vi "Door Closed Interlock Value Change.vi"(8 "error in (no error)":errorcluster, 10 "Door Closed Interlock":bool, 11 "Doors Open in":refnum<class "Doors Open.lvclass">) -> (0 "error out":errorcluster, 3 "Doors Open out":refnum<class "Doors Open.lvclass">)   [LabVIEW 2020, in "Door Controller.lvlib" / "Doors Open.lvclass"]
uses:
  Doors Open.lvclass
  C:/Users/Thomas.McQuillan/Desktop/Elevator Door Control/Door Controller/Door Controller/Door Controller.lvclass
  Application/Application/Interlock Names.ctl
  Door Controller/Door Controller.lvclass
  Application/Application.lvlib
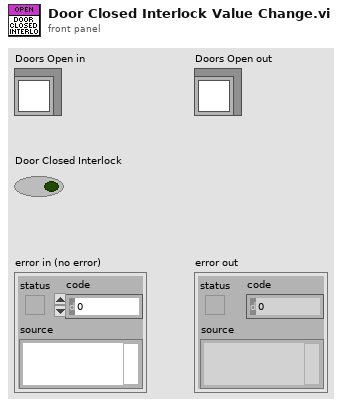
[diagram p1: front panel]
types:
  T1 = typedef "Application.lvlib/Interlock Names.ctl" = enum16{"Door Closed Interlock", "Door Open Interlock"}
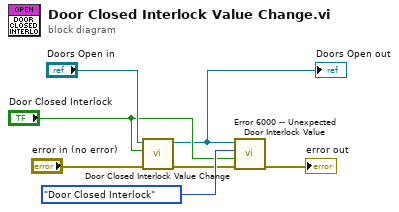
[diagram p0: block diagram]
diagram:
  n1 = call-parent "Door Closed Interlock Value Change.vi"("error in (no error)"="error in (no error)", "Door Closed Interlock"="Door Closed Interlock", "Door Controller in"="Doors Open in") -> ("error out"=w4:errorcluster, "Door Controller out"=w1:refnum<class "Doors Open.lvclass">)  [unwired: 7 in]
  "Doors Open out" <- w1
  n2 = call "Error 6000 -- Unexpected Door Interlock Value.vi"("error in (no error)"=w4, "Interlock Value"="Door Closed Interlock", "Interlock Name"=Interlock_Names."Door Closed Interlock", "Door Controller"=w1) -> ("error out"=→"error out":errorcluster)  [unwired: 7 in]
